vi "Physiological Monitor.vi"() -> ()   [LabVIEW 2020]
uses:
  Typedefs/PhysMon-Options.ctl
  Typedefs/PhysMon-Scale.ctl
  Typedefs/PhysMon-TempSensor.ctl
  Typedefs/PhysMon-HR From EKG Settings.ctl
  Typedefs/VS-Globals.vi
panel:
  out "rescale":bool
  in  "Plot what":T1={"Mode"=enum."all time", "hours"=0.1} {"hours" min=0.1 max=24.0 step=0.5}
  in  "Options":T2={"Min Interval"=0.0, "HR from ABR?"=FALSE, "HR Scale"={"Slope"=0.0, "Offset"=0.0, "Limits"={"Min"=0.0, "Max"=0.0}, "term config"=-1}, "Temp Scale"={"Slope"=0.0, "Offset"=0.0, "Limits"={"Min"=0.0, "Max"=0.0}, "term config"=-1}, "Lock?"=FALSE, "Temp Sensor"=enum."YSI", "EKG"={"Sample duration (s)"=0.0}} {"Temp Scale"."term config" items=["default"=-1, "RSE"=10083, "NRSE"=10078, "Differential"=10106, "Pseudodifferential"=12529]; "HR Scale"."term config" items=["default"=-1, "RSE"=10083, "NRSE"=10078, "Differential"=10106, "Pseudodifferential"=12529]}
  out "Temperature":dbl
  out "Heart Rate":dbl
  out "running":bool
  out "Time":string
  in  "File":path
  out "Temperature":string
  in  "Graph Toggle":bool
  out "Graph":cluster{"Graph":cluster{timestamp, dbl}[]}[](graph)
  in  "Insert Entry":bool
  in  "Entry":string
  in  "Notes":i32(listbox)
  in  "Edit Options":bool
  in  "Exit":bool
  in  "Go":bool
  out "Heart Rate":string
  in  "Abort":bool
  # "Plot..."
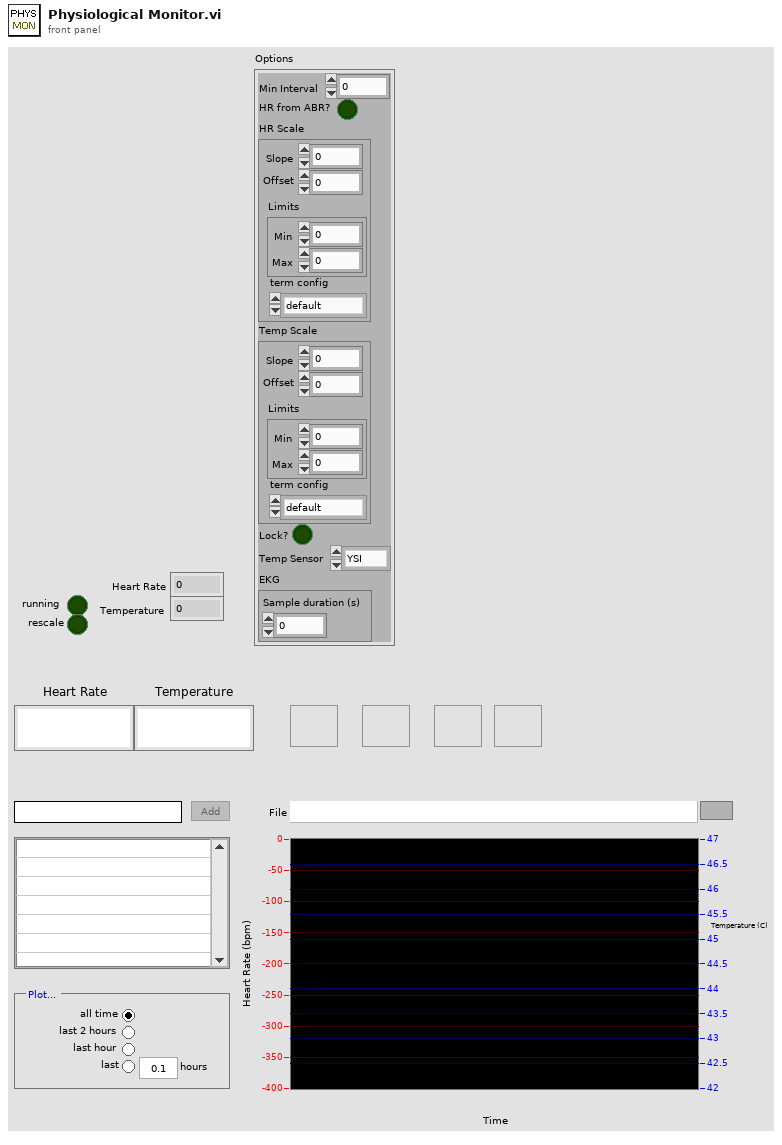
[diagram p1: front panel]
types:
  T1 = cluster{"Mode":enum32{"all time", "last 2 hours", "last hour", "last"}, "hours":dbl}
  T2 = typedef "PhysMon-Options.ctl" = cluster{"Min Interval":dbl, "HR from ABR?":bool, "HR Scale":T3, "Temp Scale":T3, "Lock?":bool, "Temp Sensor":T4, "EKG":T5}
  T3 = typedef "PhysMon-Scale.ctl" = cluster{"Slope":dbl, "Offset":dbl, "Limits":cluster{"Min":dbl, "Max":dbl}, "term config":i32}
  T4 = typedef "PhysMon-TempSensor.ctl" = enum16{"YSI", "FHC", "Custom"}
  T5 = typedef "PhysMon-HR From EKG Settings.ctl" = cluster{"Sample duration (s)":dbl}
  T6 = typedef "Semaphore RefNum" = refnum<k1>
  T7 = typedef "LVRectTypeDef.ctl" = cluster{"Left":i16, "Top":i16, "Right":i16, "Bottom":i16}
  T8 = cluster{"Timestamp":timestamp, "Heart Rate (bpm)":dbl}
  T9 = cluster{"Timestamp":timestamp, "Temperature (C)":dbl}
  T10 = cluster{"Timestamp":timestamp, "Heart Rate (bpm)":dbl}[]
  T11 = cluster{"Timestamp":timestamp, "Temperature (C)":dbl}[]
  T12 = cluster{cluster{"Timestamp":timestamp, "Heart Rate (bpm)":dbl}[]}
  T13 = cluster{cluster{"Timestamp":timestamp, "Temperature (C)":dbl}[]}
  T14 = cluster{cluster{"Timestamp":timestamp, "Temperature (C)":dbl}[]}[]
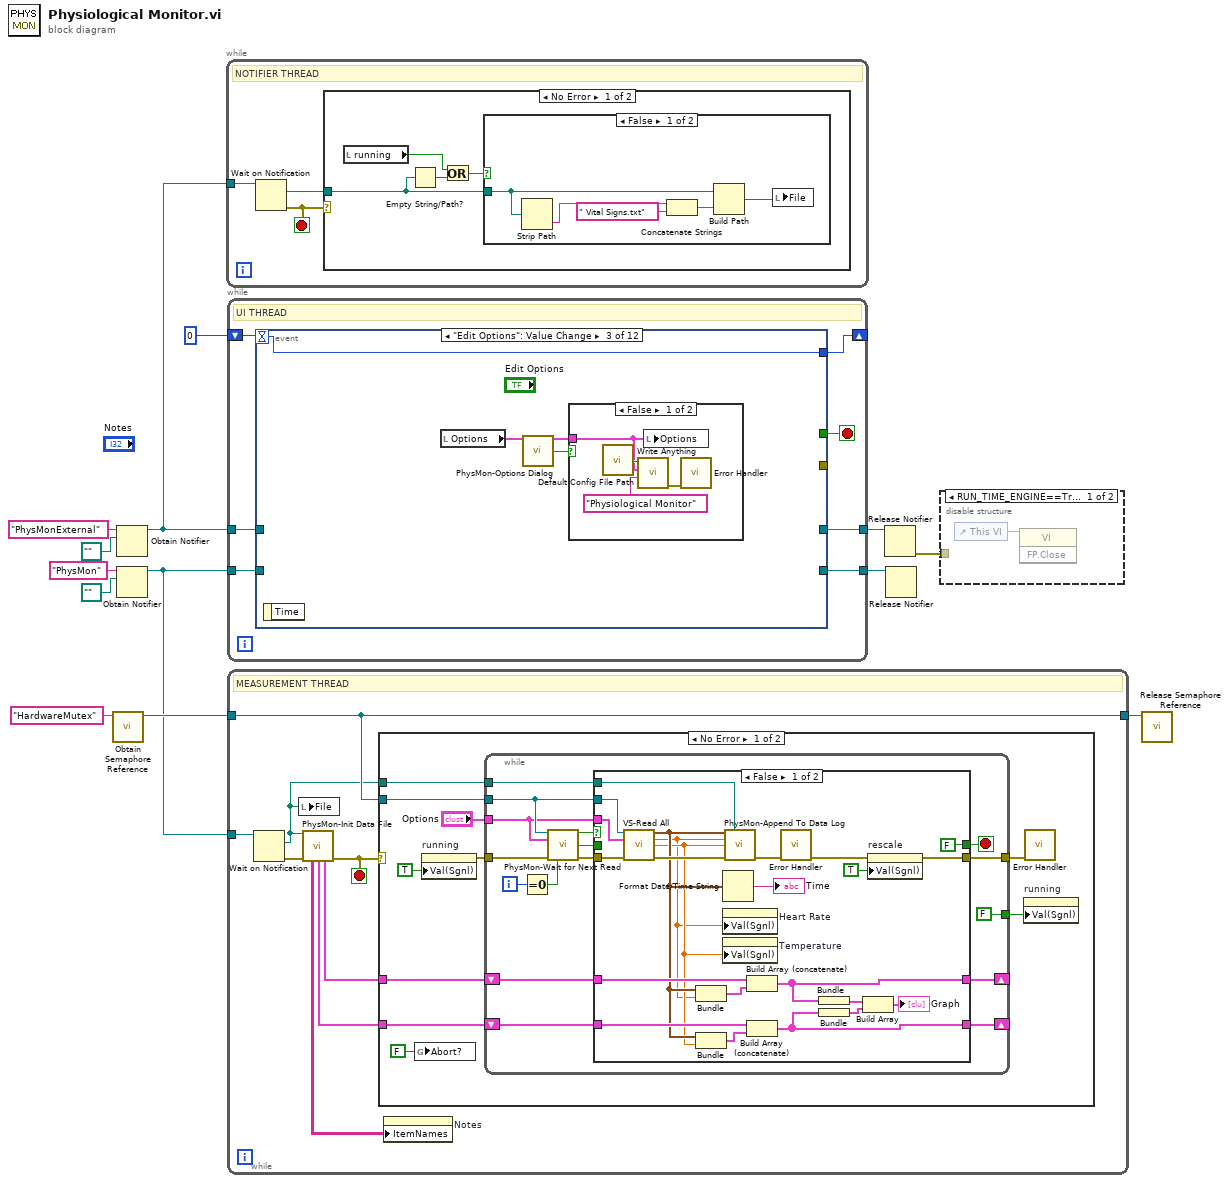
[diagram p0: block diagram]
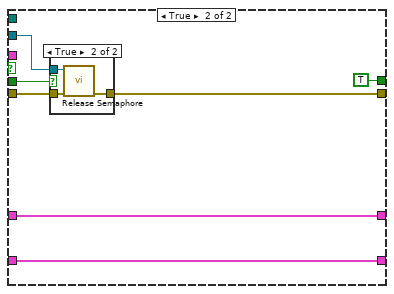
[diagram p5: hidden frame]
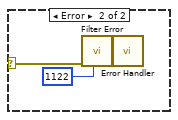
[diagram p7: hidden frame]
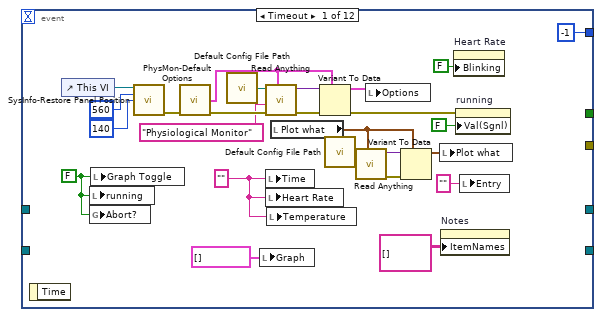
[diagram p8: hidden frame]
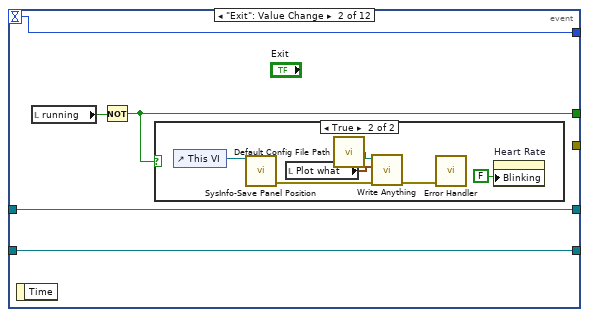
[diagram p9: hidden frame]
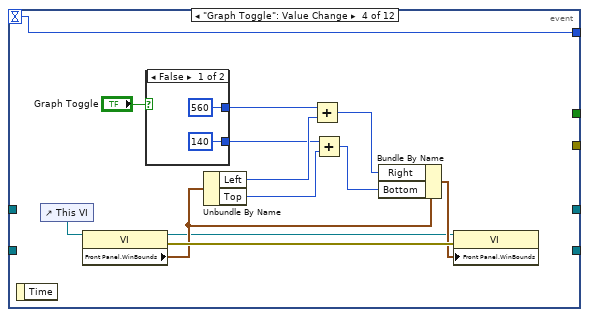
[diagram p12: hidden frame]
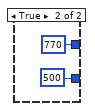
[diagram p13: hidden frame]
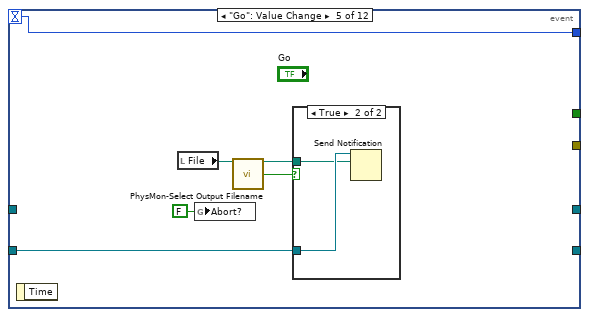
[diagram p14: hidden frame]
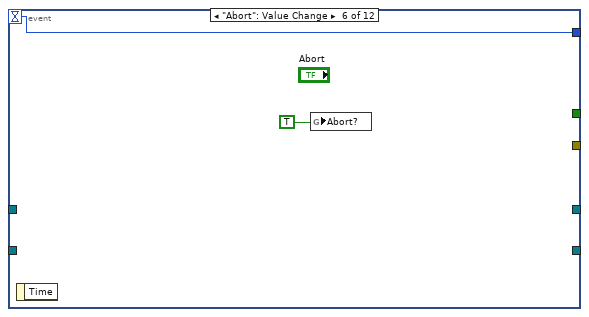
[diagram p16: hidden frame]
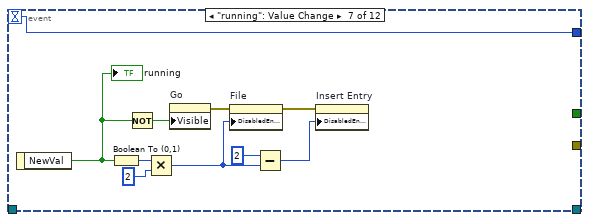
[diagram p17: hidden frame]
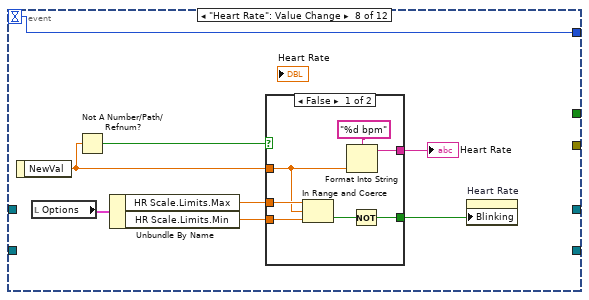
[diagram p18: hidden frame]
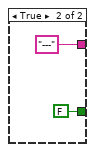
[diagram p19: hidden frame]
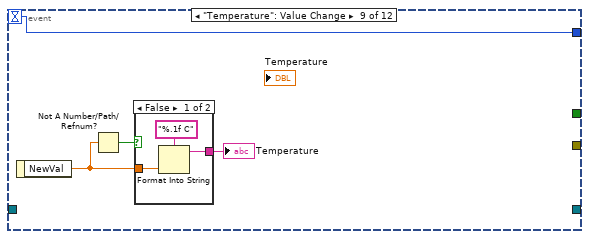
[diagram p20: hidden frame]
diagram:
  n1 = call <vilib>:"Obtain Semaphore Reference.vi"("name (unnamed)"="HardwareMutex") -> ("semaphore"=w8:T6)  [unwired: 4 in, 2 out]
  n2 = Obtain Notifier(name (unnamed)="PhysMonExternal", notification data type=path "" ("File")) -> (notifier out=w3:refnum<notifier>)  [unwired: 2 in, 2 out]
  n3 = Obtain Notifier(name (unnamed)="PhysMon", notification data type=path "" ("File")) -> (notifier out=w4:refnum<notifier>)  [unwired: 2 in, 2 out]
  n4 = while {
    tunnel: w3 -> [w16]
    stop <- w15 stop-if-true
    # "NOTIFIER THREAD"
    n5 = Wait on Notification(notifier=w16) -> (notification=w14:path, error out=w15:errorcluster)  [unwired: 3 in, 2 out]
    n6 = case shown="No Error" w15 {
      tunnel: w14 -> [w19 _]
      frame No Error {
        n7 = local read "running"() -> (w20:bool)
        n8 = Empty String/Path?(string/path=w19) -> (empty?=w17:bool)
        n9 = Or(x=w20, y=w17) -> (x .or. y?=w18:bool)
        n10 = case shown="False" w18 {
          tunnel: w19 -> [w25 _]
          frame False {
            n11 = Strip Path(path=w25) -> (name=w24:string)  [unwired: 1 out]
            n12 = Concatenate Strings(w24, " Vital Signs.txt" ("string")) -> (w22:string)
            n13 = Build Path(base path=w25, name or relative path=w22) -> (appended path=w23:path)
            n14 = local write "File"(w23) -> ()
          }
          frame True {
          }
        }
      }
      frame Error {
      }
    }
  }
  n15 = while {
    shift-right: [w31] -> _
    shift-left: 0 -> [w32]
    tunnel: w4 -> [w29]
    tunnel: [w28] -> w11
    tunnel: [w27] -> w2
    tunnel: w3 -> [w26]
    stop <- w30 stop-if-true
    # "UI THREAD"
    n16 = event shown="[2] \"Edit Options\": Value Change" {
      selector: _ -> [_ _ _ _ _ _ _ _ _ _ _ _]
      dyn-events: _ -> [_ _ _ _ _ _ _ _ _ _ _ _]
      timeout: w32 -> [_ w62 w72 w89 w99 w103 w113 w121 w134 w143 w172 w177]
      tunnel: [-1 w62 w72 w89 w99 w103 w113 w121 w134 w143 w172 w177] -> w31
      tunnel: [_ w60 _ _ _ _ _ _ _ _ _ _] -> w30
      tunnel: w29 -> [_ w59 _ _ w98 _ _ _ _ _ _ _]
      tunnel: [_ w59 _ _ _ _ _ _ _ _ _ _] -> w28
      tunnel: [_ w58 _ _ _ _ _ _ _ _ _ _] -> w27
      tunnel: w26 -> [_ w58 _ _ _ _ _ _ _ _ _ _]
      tunnel: [_ _ _ _ _ _ _ _ _ _ _ w173] -> _
      event Timeout {
        w50 = "" ("Temperature")
        w53 = FALSE ("Graph Toggle")
        n17 = event-data() -> ()  [unwired: 1 in, 1 out]
        n18 = control-ref of="This VI"() -> (w56:refnum<vi>)
        n19 = local write "running"(w53) -> ()
        n20 = global write "VS-Globals.vi" "Abort?"(w53) -> ()
        n21 = local write "Graph Toggle"(w53) -> ()
        n22 = call "SysInfo-Restore Panel Position.vi"("VI Refnum"=w56, "Width"=560, "Height"=140) -> ("error out"=w52:errorcluster)  [unwired: 10 in, 2 out]
        n23 = call "PhysMon-Default Options.vi"("error in (no error)"=w52) -> ("Options"=w42:T2, "error out"=w48:errorcluster)  [unwired: 13 in]
        n24 = call "Default Config File Path.vi"() -> ("Default config file name"=w46:path)
        n25 = local write "Graph"(cluster{"Graph":cluster{timestamp, dbl}[]}[] [] ("Graph")) -> ()
        n26 = call "Read Anything.vi"("Type of Anything"=w42, "Error In"=w48, "Section Name (Name of \"Type of Anything\")"="Physiological Monitor" ("Section Name (Name of \"Type of Anything\")"), "Path (dialog)"=w46) -> ("Error Out"=w47:errorcluster, "Anything"=w43:variant)  [unwired: 5 in, 1 out]
        n27 = local write "Time"(w50) -> ()
        n28 = local write "Heart Rate"(w50) -> ()
        n29 = local write "Temperature"(w50) -> ()
        n30 = local read "Plot what"() -> (w33:T1)
        n31 = Variant To Data(error in=w47, type=w42, Variant=w43) -> (data=w41:T2, error out=w44:errorcluster)
        n32 = call "Default Config File Path.vi"() -> ("Default config file name"=w37:path)
        n33 = call "Read Anything.vi"("Type of Anything"=w33, "Path (dialog)"=w37) -> ("Error Out"=w35:errorcluster, "Anything"=w36:variant)  [unwired: 7 in, 1 out]
        n34 = local write "Options"(w41) -> ()
        n35 = Variant To Data(error in=w35, type=w33, Variant=w36) -> (data=w34:T1)  [unwired: 1 out]
        n36 = local write "Plot what"(w34) -> ()
        n37 = property on="Notes" class="MCListbox (strict)"("ItemNames"=string[][] [] ("Item Names")) -> ()  [unwired: 2 in, 2 out]
        n38 = property on="Heart Rate" class="Str"("Blinking"=FALSE) -> ()  [unwired: 2 in, 2 out]
        n39 = property on="running" class="Bool (strict)"(error in=w44, "Val(Sgnl)"=FALSE ("Value (Signaling)")) -> ()  [unwired: 1 in, 2 out]
        n40 = local write "Entry"("" ("Entry")) -> ()
      }
      event "Exit": Value Change {
        n41 = event-data() -> ()  [unwired: 1 in, 1 out]
        n42 = local read "running"() -> (w61:bool)
        n43 = Not(x=w61) -> (.not. x?=w60:bool)
        n44 = case shown="True" w60 {
          frame False {
          }
          frame True {
            n45 = control-ref of="This VI"() -> (w68:refnum<vi>)
            n46 = call "SysInfo-Save Panel Position.vi"("VI Refnum"=w68) -> ("error out"=w65:errorcluster)  [unwired: 14 in]
            n47 = local read "Plot what"() -> (w63:T1)
            n48 = call "Default Config File Path.vi"() -> ("Default config file name"=w64:path)
            n49 = call "Write Anything.vi"("Error In"=w65, "Anything"=w63, "Path (dialog)"=w64) -> ("Error Out"=w66:errorcluster)  [unwired: 7 in, 1 out]
            n50 = call "Error Handler.vi"("error in (no error)"=w66) -> ()  [unwired: 13 in, 2 out]
            n51 = property on="Heart Rate" class="Str"("Blinking"=FALSE) -> ()  [unwired: 2 in, 2 out]
          }
        }
      }
      event "Edit Options": Value Change {
        n52 = event-data() -> ()  [unwired: 1 in, 1 out]
        n53 = local read "Options"() -> (w71:T2)
        n54 = call "PhysMon-Options Dialog.vi"("Options"=w71) -> ("Options Out"=w70:T2, "Canceled?"=w69:bool)  [unwired: 13 in]
        n55 = case shown="False" w69 {
          tunnel: w70 -> [w75 _]
          frame False {
            n56 = call "Default Config File Path.vi"() -> ("Default config file name"=w76:path)
            n57 = call "Write Anything.vi"("Section Name (Name of \"Anything\")"="Physiological Monitor" ("Section Name (Name of \"Anything\")"), "Anything"=w75, "Path (dialog)"=w76) -> ("Error Out"=w73:errorcluster)  [unwired: 7 in, 1 out]
            n58 = local write "Options"(w75) -> ()
            n59 = call "Error Handler.vi"("error in (no error)"=w73) -> ()  [unwired: 13 in, 2 out]
          }
          frame True {
          }
        }
      }
      event "Graph Toggle": Value Change {
        n60 = event-data() -> ()  [unwired: 1 in, 1 out]
        n61 = control-ref of="This VI"() -> (w80:refnum<vi>)
        n62 = property class="VI"(reference=w80) -> (reference out=w81:refnum<vi>, error out=w87:errorcluster, "Front Panel.WinBounds"=w86:T7)  [unwired: 1 in]
        n63 = case shown="False" "Graph Toggle" {
          tunnel: [560 770] -> w79
          tunnel: [140 500] -> w78
          frame False {
          }
          frame True {
          }
        }
        n64 = Unbundle By Name(w86) -> ("Left"=w82:i16, "Top"=w77:i16)
        n65 = Add(x=w79, y=w82) -> (x+y=w83:i32)
        n66 = Add(x=w78, y=w77) -> (x+y=w84:i32)
        n67 = Bundle By Name(cluster=w86, "Right"=w83, "Bottom"=w84) -> (w85:T7)
        n68 = property class="VI"(reference=w81, error in=w87, "Front Panel.WinBounds"=w85) -> ()  [unwired: 2 out]
      }
      event "Go": Value Change {
        n69 = event-data() -> ()  [unwired: 1 in, 1 out]
        n70 = local read "File"() -> (w95:path)
        n71 = global write "VS-Globals.vi" "Abort?"(FALSE ("Abort?")) -> ()
        n72 = call "PhysMon-Select Output Filename.vi"("File"=w95) -> ("File Out"=w97:path, "Continue?"=w96:bool)  [unwired: 12 in, 1 out]
        n73 = case shown="True" w96 {
          tunnel: w98 -> [_ w101]
          tunnel: w97 -> [_ w100]
          frame False {
          }
          frame True {
            n74 = Send Notification(notification=w100, notifier=w101) -> ()  [unwired: 1 in, 2 out]
          }
        }
      }
      event "Abort": Value Change {
        n75 = event-data() -> ()  [unwired: 1 in, 1 out]
        n76 = global write "VS-Globals.vi" "Abort?"(TRUE ("abort")) -> ()
      }
      event "running": Value Change {
        n77 = event-data() -> ("NewVal"=w111:bool)  [unwired: 1 in]
        "running" <- w111
        n78 = Boolean To (0,1)(Boolean=w111) -> (0, 1=w110:i16)
        n79 = Not(x=w111) -> (.not. x?=w112:bool)
        n80 = Multiply(x=w110, y=i16 2) -> (x*y=w106:i16)
        n81 = property on="Go" class="Bool"("Visible"=w112) -> (error out=w108:errorcluster)  [unwired: 2 in, 1 out]
        n82 = property on="File" class="Path"(error in=w108, "DisabledEnum"=w106) -> (error out=w107:errorcluster)  [unwired: 1 in, 1 out]
        n83 = Subtract(x=i16 2, y=w106) -> (x-y=w104:i16)
        n84 = property on="Insert Entry" class="Bool"(error in=w107, "DisabledEnum"=w104) -> ()  [unwired: 1 in, 2 out]
      }
      event "Heart Rate": Value Change {
        n85 = event-data() -> ("NewVal"=w118:dbl)  [unwired: 1 in]
        n86 = local read "Options"() -> (w117:T2)
        n87 = Not A Number/Path/Refnum?(number/path/refnum=w118) -> (NaN/Path/Refnum?=w119:bool)
        n88 = Unbundle By Name(w117) -> ("HR Scale.Limits.Max"=w116:dbl, "HR Scale.Limits.Min"=w115:dbl)
        n89 = case shown="False" w119 {
          tunnel: [w128 "---"] -> w120
          tunnel: w118 -> [w124 _]
          tunnel: w116 -> [w126 _]
          tunnel: w115 -> [w125 _]
          tunnel: [w122 FALSE] -> w114
          frame False {
            n90 = In Range and Coerce(upper limit=w126, x=w124, lower limit=w125) -> (In Range?=w123:bool)  [unwired: 1 out]
            n91 = Format Into String(format string="%d bpm", w124) -> (resulting string=w128:string)  [unwired: 2 in, 1 out]
            n92 = Not(x=w123) -> (.not. x?=w122:bool)
          }
          frame True {
          }
        }
        "Heart Rate" <- w120
        n93 = property on="Heart Rate" class="Str"("Blinking"=w114) -> ()  [unwired: 2 in, 2 out]
      }
      event "Temperature": Value Change {
        n94 = event-data() -> ("NewVal"=w132:dbl)  [unwired: 1 in]
        n95 = Not A Number/Path/Refnum?(number/path/refnum=w132) -> (NaN/Path/Refnum?=w131:bool)
        n96 = case shown="False" w131 {
          tunnel: [w137 "---"] -> w133
          tunnel: w132 -> [w135 _]
          frame False {
            n97 = Format Into String(format string="%.1f C", w135) -> (resulting string=w137:string)  [unwired: 2 in, 1 out]
          }
          frame True {
          }
        }
        "Temperature" <- w133
      }
      event "File": Value Change {
        n98 = event-data() -> ()  [unwired: 1 in, 1 out]
        n99 = call "PhysMon-Read Data Log.vi"("Path"="File") -> ("Notes"=w139:string[][], "Vital Signs Graph"=w140:cluster{"HR Data":cluster{timestamp, dbl}[]}[], "error out"=w141:errorcluster)  [unwired: 12 in]
        n100 = case shown="No Error" w141 {
          selector: w141 -> [_ w161]
          tunnel: w140 -> [w160 _]
          tunnel: w139 -> [w145 _]
          frame No Error {
            n101 = Index Array(array=w160) -> (element #1=w158:cluster{"HR Data":cluster{timestamp, dbl}[]}, element #2=w147:cluster{"HR Data":cluster{timestamp, dbl}[]})  [unwired: 2 in]
            n102 = local write "Graph"(w160) -> ()
            n103 = Unbundle(w158) -> ("HR Data"=w157:cluster{timestamp, dbl}[])
            n104 = Unbundle(w147) -> ("HR Data"=w150:cluster{timestamp, dbl}[])
            n105 = Array Size(array=w157) -> (size(s)=w159:i32)
            n106 = Array Size(array=w150) -> (size(s)=w151:i32)
            n107 = property on="rescale" class="Bool (strict)"("Val(Sgnl)"=TRUE ("Value (Signaling)")) -> ()  [unwired: 2 in, 2 out]
            n108 = Decrement(x=w159) -> (x-1=w156:i32)
            n109 = Decrement(x=w151) -> (x-1=w149:i32)
            n110 = Index Array(array=w157, index=w156) -> (element=w155:cluster{timestamp, dbl})
            n111 = Index Array(array=w150, index=w149) -> (element=w148:cluster{timestamp, dbl})
            n112 = property on="Notes" class="MCListbox (strict)"("ItemNames"=w145) -> ()  [unwired: 2 in, 2 out]
            n113 = Unbundle(w155) -> (w154:timestamp, w152:dbl)
            n114 = Unbundle(w148) -> (w146:dbl)  [unwired: 1 out]
            n115 = Format Date/Time String(seconds (now)=w154) -> (date/time string=w153:string)  [unwired: 2 in]
            n116 = property on="Heart Rate" class="DigNum (strict)"("Val(Sgnl)"=w152) -> ()  [unwired: 2 in, 2 out]
            n117 = property on="Temperature" class="DigNum (strict)"("Val(Sgnl)"=w146) -> ()  [unwired: 2 in, 2 out]
            n118 = local write "Time"(w153) -> ()
          }
          frame Error {
            n119 = call "Error Handler.vi"("error in (no error)"=w161) -> ()  [unwired: 13 in, 2 out]
          }
        }
      }
      event "Insert Entry": Value Change {
        n120 = event-data() -> ()  [unwired: 1 in, 1 out]
        n121 = property on="Notes" class="MCListbox (strict)"() -> ("ItemNames"=w169:string[][])  [unwired: 2 in, 2 out]
        n122 = Get Date/Time In Seconds() -> (seconds since 1Jan1904=w165:timestamp)
        n123 = Format Date/Time String(time format string (%c)="%H:%M:%S", seconds (now)=w165) -> (date/time string=w170:string)  [unwired: 1 in]
        n124 = local read "File"() -> (w166:path)
        n125 = Build Array(w170, "Entry") -> (w168:string[])
        n126 = Build Array (concatenate)(w169, w168) -> (w167:string[][])
        n127 = call "PhysMon-Append To Data Log.vi"("Timestamp"=w165, "Path"=w166, "Note"="Entry") -> ("error out"=w163:errorcluster)  [unwired: 12 in]
        n128 = property on="Notes" class="MCListbox (strict)"("ItemNames"=w167) -> ()  [unwired: 2 in, 2 out]
        n129 = property on="Entry" class="Str"(error in=w163, "Value"="" ("Entry")) -> ()  [unwired: 1 in, 2 out]
      }
      event "Plot what", "rescale": Value Change {
        n130 = event-data() -> ()  [unwired: 1 in, 1 out]
        n131 = local read "running"() -> (w174:bool)
        n132 = control-ref of="Graph"() -> (w176:refnum<vi>)
        n133 = call "VS-Scale Time Axis.vi"("Graph Ref"=w176, "Running?"=w174, "Plot what"="Plot what") -> ("error out"=w173:errorcluster)  [unwired: 12 in]
      }
    }
  }
  n134 = while {
    tunnel: w4 -> [w185]
    tunnel: w8 -> [w180]
    tunnel: [w180] -> w7
    stop <- w183 stop-if-true
    # "MEASUREMENT THREAD"
    n135 = Wait on Notification(notifier=w185) -> (notification=w179:path, error out=w184:errorcluster)  [unwired: 3 in, 2 out]
    n136 = local write "File"(w179) -> ()
    n137 = call "PhysMon-Init Data File.vi"("Path"=w179, "error in (no error)"=w184) -> ("Notes"=w178:string[][], "Temp Data"=w181:cluster{timestamp, dbl}[], "HR Data"=w182:cluster{timestamp, dbl}[], "error out"=w183:errorcluster)  [unwired: 10 in]
    n138 = case shown="No Error" w183 {
      selector: w183 -> [_ w248]
      tunnel: w179 -> [w192 _]
      tunnel: w182 -> [w187 _]
      tunnel: w181 -> [w186 _]
      tunnel: w180 -> [w188 _]
      frame No Error {
        n139 = global write "VS-Globals.vi" "Abort?"(FALSE ("Abort?")) -> ()
        n140 = property on="running" class="Bool (strict)"("Val(Sgnl)"=TRUE ("Value (Signaling)")) -> (error out=w194:errorcluster)  [unwired: 2 in, 1 out]
        n141 = while {
          tunnel: w194 -> [w205]
          tunnel: [w201] -> w189
          shift-right: [w208] -> _
          shift-left: w187 -> [w211]
          shift-right: [w207] -> _
          shift-left: w186 -> [w210]
          tunnel: w192 -> [w209]
          tunnel: "Options" -> [w199]
          tunnel: [FALSE ("Value (Signaling)")] -> w190
          tunnel: w188 -> [w200]
          i -> [w198]
          stop <- w202 stop-if-true
          n142 = Equal To 0?(x=w198) -> (x = 0?=w197:bool)
          n143 = call "PhysMon-Wait for Next Read.vi"("Hardware Mutex"=w200, "Options"=w199, "Error"=w205, "First Call?"=w197) -> ("Stop?"=w203:bool, "Mutex Acquired"=w196:bool, "Error Out"=w204:errorcluster)  [unwired: 9 in]
          n144 = case shown="False" w203 {
            tunnel: w211 -> [w234 w241]
            tunnel: w210 -> [w233 w240]
            tunnel: w209 -> [w231 _]
            tunnel: [w230 w241] -> w208
            tunnel: [w229 w240] -> w207
            tunnel: w199 -> [w222 _]
            tunnel: w204 -> [w224 w238]
            tunnel: [FALSE TRUE] -> w202
            tunnel: w200 -> [w221 w237]
            tunnel: [w215 w236] -> w201
            tunnel: w196 -> [_ w235]
            frame False {
              n145 = call "VS-Read All.vi"("Hardware Mutex"=w221, "Options"=w222, "error in (no error)"=w224) -> ("Timestamp"=w228:timestamp, "Heart Rate (bpm)"=w225:dbl, "Temperature (C)"=w226:dbl, "error out"=w232:errorcluster)  [unwired: 9 in]
              n146 = Bundle("Timestamp"=w228, "Heart Rate (bpm)"=w225) -> (w220:T8)  [unwired: 1 in]
              n147 = Bundle("Timestamp"=w228, "Temperature (C)"=w226) -> (w219:T9)  [unwired: 1 in]
              n148 = Format Date/Time String(seconds (now)=w228) -> (date/time string=→"Time":string)  [unwired: 2 in]
              n149 = property on="Heart Rate" class="DigNum (strict)"("Val(Sgnl)"=w225) -> ()  [unwired: 2 in, 2 out]
              n150 = property on="Temperature" class="DigNum (strict)"("Val(Sgnl)"=w226) -> ()  [unwired: 2 in, 2 out]
              n151 = call "PhysMon-Append To Data Log.vi"("Timestamp"=w228, "Path"=w231, "Heart Rate (bpm)"=w225, "Temperature (C)"=w226, "error in (no error)"=w232) -> ("error out"=w213:errorcluster)  [unwired: 10 in]
              n152 = Build Array (concatenate)(w234, w220) -> (w230:T10)
              n153 = Build Array (concatenate)(w233, w219) -> (w229:T11)
              n154 = call "Error Handler.vi"("error in (no error)"=w213) -> ("No Error"=w212:errorcluster)  [unwired: 13 in, 1 out]
              n155 = Bundle(w230) -> (w217:T12)  [unwired: 1 in]
              n156 = Bundle(w229) -> (w216:T13)  [unwired: 1 in]
              n157 = Build Array(w217, w216) -> (→"Graph":T14)
              n158 = property on="rescale" class="Bool (strict)"(error in=w212, "Val(Sgnl)"=TRUE ("Value (Signaling)")) -> (error out=w215:errorcluster)  [unwired: 1 in, 1 out]
            }
            frame True {
              n159 = case shown="True" w235 {
                tunnel: w238 -> [w242 w245]
                tunnel: w237 -> [_ w244]
                tunnel: [w242 w243] -> w236
                frame False {
                }
                frame True {
                  n160 = call <vilib>:"Release Semaphore.vi"("error in (no error)"=w245, "semaphore"=w244) -> ("error out"=w243:errorcluster)  [unwired: 4 in, 1 out]
                }
              }
            }
          }
        }
        n161 = property on="running" class="Bool (strict)"("Val(Sgnl)"=w190) -> ()  [unwired: 2 in, 2 out]
        n162 = call "Error Handler.vi"("error in (no error)"=w189) -> ()  [unwired: 13 in, 2 out]
      }
      frame Error {
        n163 = call "Filter Error.vi"("error in (no error)"=w248, "code to ignore"=1122) -> ("error out"=w247:errorcluster)  [unwired: 9 in]
        n164 = call "Error Handler.vi"("error in (no error)"=w247) -> ()  [unwired: 13 in, 2 out]
      }
    }
    n165 = property on="Notes" class="MCListbox (strict)"("ItemNames"=w178) -> ()  [unwired: 2 in, 2 out]
  }
  n166 = Release Notifier(notifier=w2) -> (error out=w1:errorcluster)  [unwired: 2 in, 2 out]
  n167 = Release Notifier(notifier=w11) -> ()  [unwired: 2 in, 3 out]
  n168 = disable-structure shown="RUN_TIME_ENGINE==True" {
    disable-tunnel: w1 -> [_ _]
    frame condition #0 {
      n169 = control-ref of="This VI"() -> (w249:refnum<vi>)
      n170 = invoke class="VI" method="FP.Close"(reference=w249) -> ()  [unwired: 2 in, 3 out]
    }
    frame condition #1 (active) {
    }
  }
  n171 = call <vilib>:"Release Semaphore Reference.vi"("semaphore"=w7) -> ()  [unwired: 9 in, 2 out]
